vi "Manual profile generator.vi"() -> ()   [LabVIEW 2017, in "labview-standard-library.lvlib" / "automode-scripting.lvlib"]
uses:
  automode-scripting.lvlib
  Motion_Profile_Inputs.ctl
  Motion_Profile_Outputs.ctl
panel:
  out "Motion profile outputs":T1
  in  "Motion profile inputs":T2={"Max Acceleration (inches/sec^2)"=0.0, "Maximun Speed (IPS)"=0.0, "Control loop Hz"=100.0, "Distance in inches"=0.0, "Max \"Jerk\" (inches/sec^3)"=0.0}
  in  "Generate Profile?":bool
  in  "stop":bool
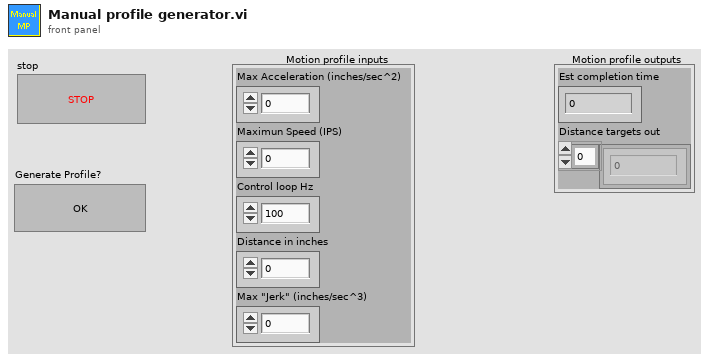
[diagram p1: front panel]
types:
  T1 = typedef "labview-standard-library.lvlib/automode-scripting.lvlib/Motion_Profile_Outputs.ctl" = cluster{"Est completion time":dbl, "Distance targets out":dbl[]}
  T2 = typedef "labview-standard-library.lvlib/automode-scripting.lvlib/Motion_Profile_Inputs.ctl" = cluster{"Max Acceleration (inches/sec^2)":dbl, "Maximun Speed (IPS)":dbl, "Control loop Hz":dbl, "Distance in inches":dbl, "Max \"Jerk\" (inches/sec^3)":dbl}
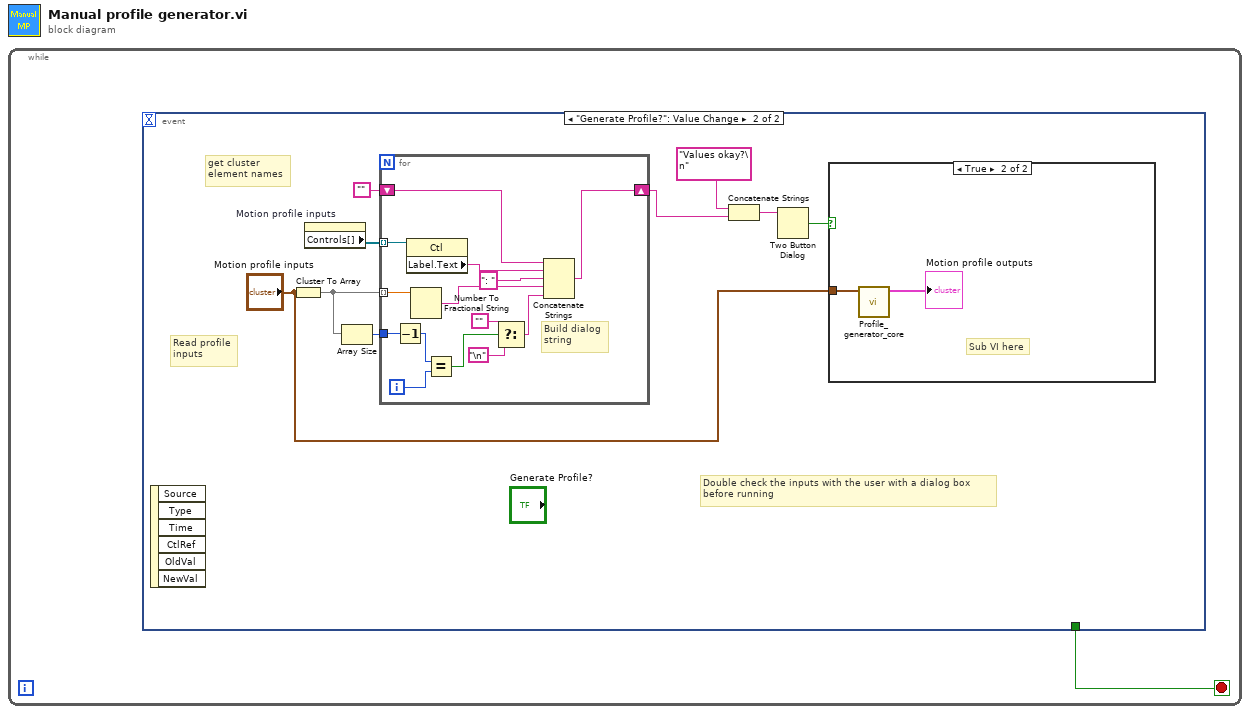
[diagram p0: block diagram]
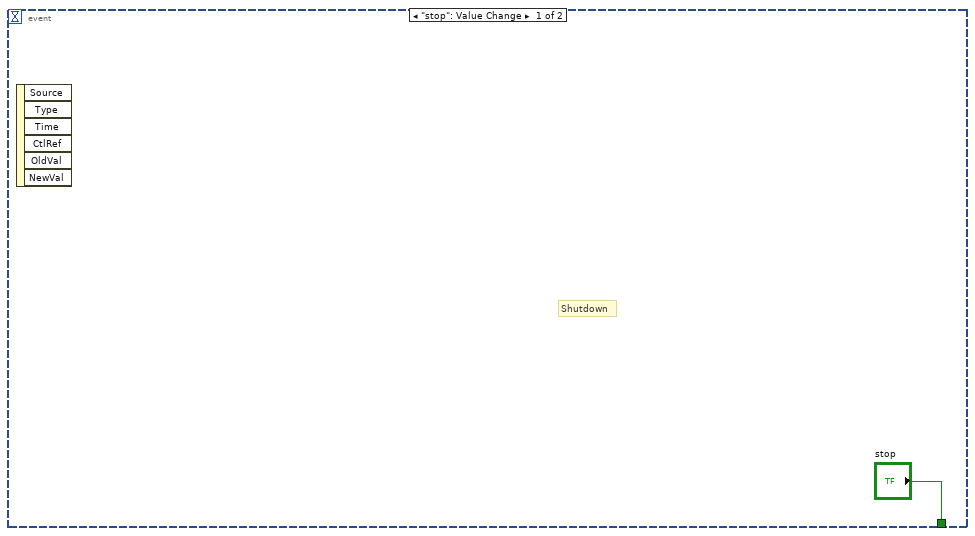
[diagram p2: hidden frame]
diagram:
  n1 = while {
    stop <- w1 stop-if-true
    n2 = event shown="[1] \"Generate Profile?\": Value Change" {
      selector: _ -> [_ _]
      dyn-events: _ -> [_ _]
      timeout: _ -> [_ _]
      tunnel: ["stop" _] -> w1
      event "stop": Value Change {
        # "Shutdown"
        n3 = event-data() -> ()  [unwired: 1 in, 6 out]
      }
      event "Generate Profile?": Value Change {
        # "get cluster\nelement names"
        # "Read profile\ninputs"
        # "Double check the inputs with the user with a dialog box\nbefore running"
        n4 = event-data() -> ()  [unwired: 1 in, 6 out]
        n5 = Cluster To Array(cluster="Motion profile inputs") -> (array=w7:dbl[])
        n6 = property on="Motion profile inputs" class="Clust (strict)"() -> ("Controls[]"=w10:refnum<vi>[])  [unwired: 2 in, 2 out]
        n7 = Array Size(array=w7) -> (size(s)=w8:i32)
        n8 = for {
          tunnel: w7 -> [w26] mode=indexing
          tunnel: w10 -> [w27] mode=indexing
          shift-right: [w22] -> w5
          shift-left: "" -> [w21]
          tunnel: w8 -> [w20]
          i -> [w18]
          # "Build dialog\nstring"
          n9 = Decrement(x=w20) -> (x-1=w17:i32)
          n10 = property class="Ctl"(reference=w27) -> ("Label.Text"=w25:string)  [unwired: 1 in, 2 out]
          n11 = Number To Fractional String(number=w26) -> (F-format string=w23:string)  [unwired: 3 in]
          n12 = Equal?(x=w17, y=w18) -> (x = y?=w16:bool)
          n13 = Select(t="", s=w16, f="\n") -> (s? t:f=w19:string)
          n14 = Concatenate Strings(w21, w25, ": " ("string"), w23, w19) -> (w22:string)
        }
        n15 = Concatenate Strings("Values okay?\n" ("string"), w5) -> (w11:string)
        n16 = Two Button Dialog(message=w11) -> (T button?=w4:bool)  [unwired: 2 in]
        n17 = case shown="True" w4 {
          tunnel: "Motion profile inputs" -> [_ w13]
          frame False {
          }
          frame True {
            # "Sub VI here"
            n18 = call "Profile_generator_core.vi"("Motion profile inputs"=w13) -> ("Motion profile outputs"=→"Motion profile outputs":T1)  [unwired: 10 in]
          }
        }
      }
    }
  }
